vi "Write Update Mode.vi"(8 "error in (no error)":errorcluster, 10 "UpdateMode":u8, 11 "IntensityChart.lvclass in":refnum<class "IntensityChart.lvclass">) -> (0 "error out":errorcluster, 3 "IntensityChart.lvclass out":refnum<class "IntensityChart.lvclass">)   [LabVIEW 2015, in "IntensityChart.lvclass"]
uses:
  IntensityChart.lvclass
  IntensityChart.lvclass/IntensityChart.ctl
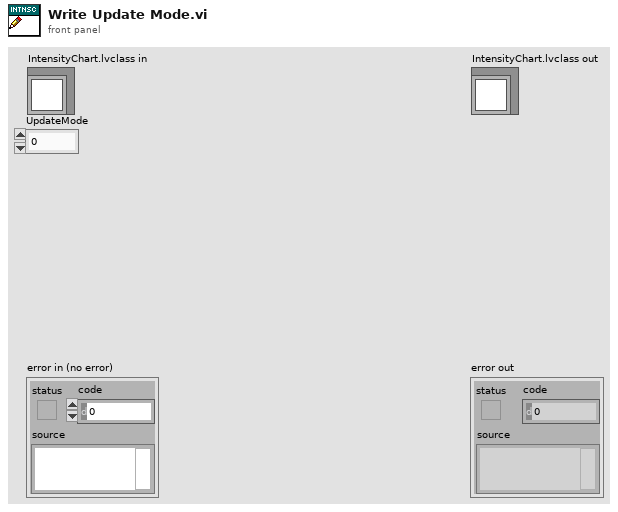
[diagram p1: front panel]
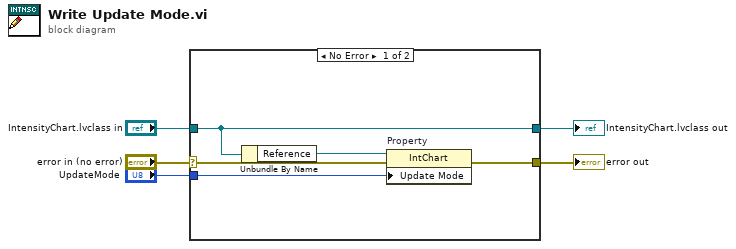
[diagram p0: block diagram]
diagram:
  n1 = case shown="No Error" "error in (no error)" {
    selector: "error in (no error)" -> [w6 w12]
    tunnel: [w10 w12] -> w4
    tunnel: [w8 w11] -> w2
    tunnel: "IntensityChart.lvclass in" -> [w8 w11]
    tunnel: "UpdateMode" -> [w9 _]
    frame No Error {
      n2 = Unbundle By Name(w8) -> ("Reference"=w7:refnum<vi>)
      n3 = property on="Property" class="IntChart"(reference=w7, error in=w6, "Update Mode"=w9) -> (error out=w10:errorcluster)  [unwired: 1 out]
    }
    frame Error {
    }
  }
  "error out" <- w4
  "IntensityChart.lvclass out" <- w2
